vi "Reentrant.vi"() -> ()   [LabVIEW 2011]
uses:
  GlobalStop.vi
panel:
  in  "Cluster":cluster{"Machine":string, "Port":u16}={"Machine"="localhost", "Port"=0}
  out "Data Received":string
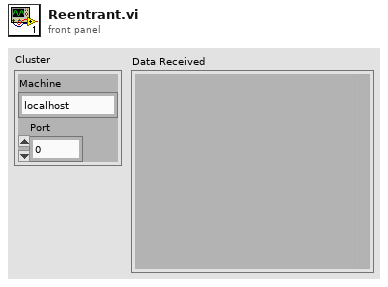
[diagram p1: front panel]
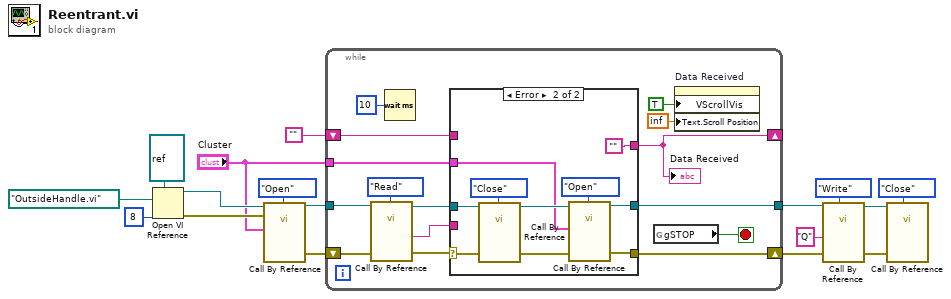
[diagram p0: block diagram]
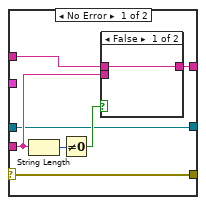
[diagram p2: hidden frame]
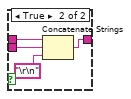
[diagram p3: hidden frame]
diagram:
  n1 = Open VI Reference(type specifier VI Refnum (for type only)=refnum<vi> refnum, vi path=path "OutsideHandle.vi", options=8) -> (vi reference=w14:refnum<vi>, error out=w12:errorcluster)  [unwired: 3 in]
  n2 = call-by-ref "?"(reference=w14, error in=w12, "Mode"=enum16{"Open", "Read", "Write", "Close"}."Open", "Cluster"="Cluster") -> (reference out=w5:refnum<vi>, "error out"=w10:errorcluster)  [unwired: 8 in, 2 out]
  n3 = while {
    shift-right: [w31] -> w8
    shift-left: w10 -> [w24]
    shift-right: [w28] -> _
    shift-left: "" -> [w30]
    tunnel: "Cluster" -> [w29]
    tunnel: w5 -> [w20]
    tunnel: [w19] -> w4
    stop <- w18 stop-if-true
    n4 = call-by-ref "?"(reference=w20, "Mode"=enum16{"Open", "Read", "Write", "Close"}."Read", "error in (no error)"=w24) -> (reference out=w21:refnum<vi>, "error out"=w23:errorcluster, "data out"=w22:string)  [unwired: 9 in, 1 out]
    n5 = Wait (ms)(milliseconds to wait=u32 10) -> ()  [unwired: 1 out]
    n6 = case shown="Error" w23 {
      selector: w23 -> [w39 w52]
      tunnel: [w39 w49] -> w31
      tunnel: w22 -> [w35 _]
      tunnel: w30 -> [w36 _]
      tunnel: [w34 ""] -> w28
      tunnel: w29 -> [_ w45]
      tunnel: w21 -> [w33 w48]
      tunnel: [w33 w46] -> w19
      frame No Error {
        n7 = String Length(string=w35) -> (length=w38:i32)
        n8 = Not Equal To 0?(x=w38) -> (x != 0?=w37:bool)
        n9 = case shown="False" w37 {
          tunnel: w36 -> [w40 w44]
          tunnel: w35 -> [_ w42]
          tunnel: [w40 w43] -> w34
          frame False {
          }
          frame True {
            n10 = Concatenate Strings(w44, w42, "\r\n" ("Substring")) -> (w43:string)
          }
        }
      }
      frame Error {
        n11 = call-by-ref "?"(reference=w48, "Mode"=enum16{"Open", "Read", "Write", "Close"}."Close", "error in (no error)"=w52) -> (reference out=w47:refnum<vi>, "error out"=w50:errorcluster)  [unwired: 9 in, 2 out]
        n12 = call-by-ref "?"(reference=w47, "Mode"=enum16{"Open", "Read", "Write", "Close"}."Open", "error in (no error)"=w50, "Cluster"=w45) -> (reference out=w46:refnum<vi>, "error out"=w49:errorcluster)  [unwired: 8 in, 2 out]
      }
    }
    "Data Received" <- w28
    n13 = global read "GlobalStop.vi" "gSTOP"() -> (w18:bool)
    n14 = property on="Data Received" class="Str"("VScrollVis"=TRUE ("Vertical Scrollbar Visible"), "Text.Scroll Position"=inf) -> ()  [unwired: 2 in, 2 out]
  }
  n15 = call-by-ref "?"(reference=w4, "Mode"=enum16{"Open", "Read", "Write", "Close"}."Write", "error in (no error)"=w8, "data in"="Q") -> (reference out=w3:refnum<vi>, "error out"=w6:errorcluster)  [unwired: 8 in, 2 out]
  n16 = call-by-ref "?"(reference=w3, "Mode"=enum16{"Open", "Read", "Write", "Close"}."Close", "error in (no error)"=w6) -> ()  [unwired: 9 in, 4 out]
